vi "input.vi"(2 "位数(2)":i32=2, 3 "in":dbl=1.2345) -> (0 "out":dbl format="%.6f", 1 "值改变?":bool)   [LabVIEW 2018]
panel:
  in  "ESC":bool
  in  "C":bool
  in  "字符串":string
  in  ".":bool
  in  "0":bool
  in  "-":bool
  in  "bk":bool
  in  "en":bool
  in  "3":bool
  in  "2":bool
  in  "1":bool
  in  "6":bool
  in  "5":bool
  in  "4":bool
  in  "9":bool
  in  "8":bool
  in  "7":bool
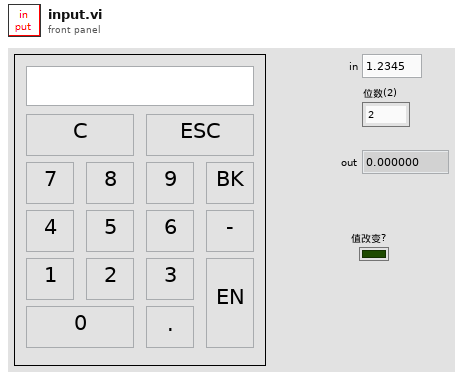
[diagram p1: front panel]
types:
  T1 = enum8{"Enabled", "Disabled", "Disabled and Grayed Out"}
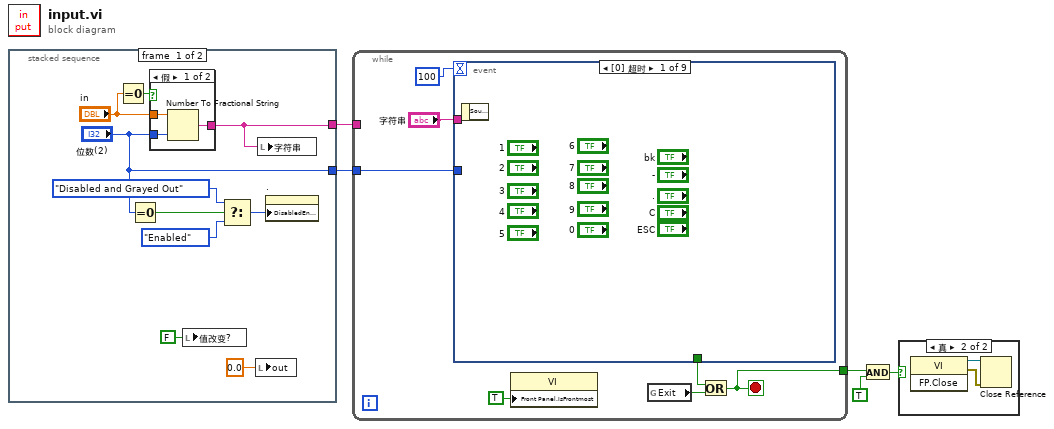
[diagram p0: block diagram]
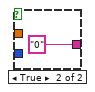
[diagram p2: hidden frame]
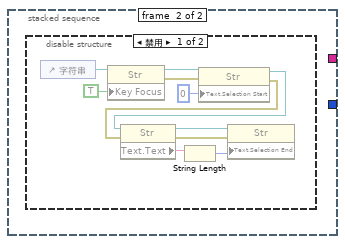
[diagram p3: hidden frame]
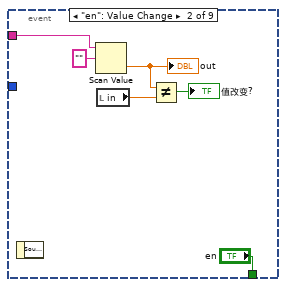
[diagram p6: hidden frame]
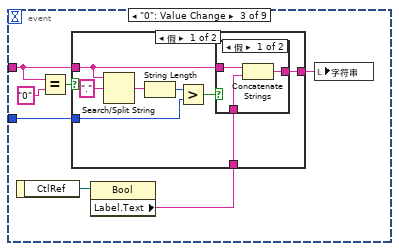
[diagram p7: hidden frame]
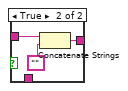
[diagram p8: hidden frame]
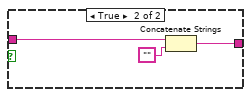
[diagram p9: hidden frame]
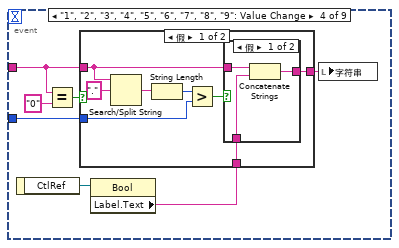
[diagram p10: hidden frame]
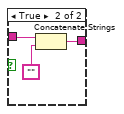
[diagram p11: hidden frame]
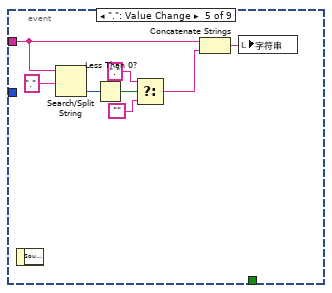
[diagram p13: hidden frame]
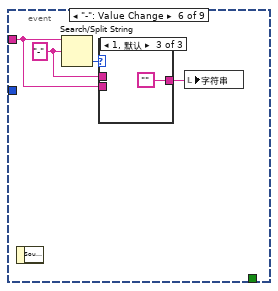
[diagram p14: hidden frame]
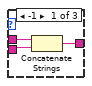
[diagram p15: hidden frame]
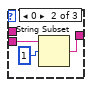
[diagram p16: hidden frame]
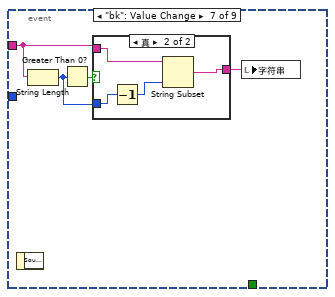
[diagram p17: hidden frame]
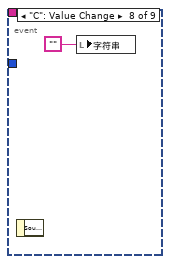
[diagram p19: hidden frame]
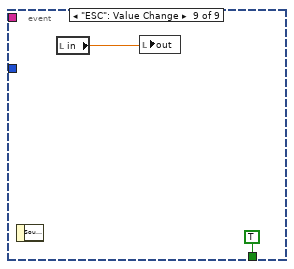
[diagram p20: hidden frame]
diagram:
  n1 = stacked-sequence {
    tunnel: [w15 _] -> w5
    tunnel: ["位数(2)" _] -> w1
    frame #0 {
      n2 = Equal To 0?(x="in") -> (x = 0?=w13:bool)
      n3 = Equal To 0?(x="位数(2)") -> (x = 0?=w9:bool)
      n4 = case shown="假" w13 {
        tunnel: "in" -> [w18 _]
        tunnel: [w17 "0"] -> w15
        tunnel: "位数(2)" -> [w16 _]
        frame False {
          n5 = Number To Fractional String(number=w18, precision (6)=w16) -> (F-format string=w17:string)  [unwired: 2 in]
        }
        frame True {
        }
      }
      n6 = local write "值改变?"(FALSE ("值改变")) -> ()
      n7 = Select(t=T1."Disabled and Grayed Out" ("禁用"), s=w9, f=T1."Enabled" ("禁用")) -> (s? t:f=w8:T1)
      n8 = local write "out"(0.0) -> ()
      n9 = local write "字符串"(w15) -> ()
      n10 = property on="." class="Bool"("DisabledEnum"=w8) -> ()  [unwired: 2 in, 2 out]
    }
    frame #1 {
      n11 = disable-structure shown="禁用" {
        frame Disabled {
          n12 = control-ref of="字符串"() -> (w28:refnum<vi>)
          n13 = property class="Str"(reference=w28, "Key Focus"=TRUE ("键选中")) -> (reference out=w25:refnum<vi>, error out=w24:errorcluster)  [unwired: 1 in]
          n14 = property class="Str"(reference=w25, error in=w24, "Text.Selection Start"=u32 0 ("文本.选择区域:起始")) -> (reference out=w21:refnum<vi>, error out=w22:errorcluster)
          n15 = property class="Str"(reference=w21, error in=w22) -> (reference out=w29:refnum<vi>, error out=w20:errorcluster, "Text.Text"=w30:string)
          n16 = String Length(string=w30) -> (length=w26:i32)
          n17 = property class="Str"(reference=w29, error in=w20, "Text.Selection End"=w26) -> ()  [unwired: 2 out]
        }
        frame Enabled {
        }
      }
    }
  }
  n18 = while {
    tunnel: [w34] -> w4
    tunnel: w5 -> [_]
    tunnel: w1 -> [w31]
    stop <- w34 stop-if-true
    n19 = event shown="[0] 超时" {
      selector: _ -> [_ _ _ _ _ _ _ _ _]
      dyn-events: _ -> [_ _ _ _ _ _ _ _ _]
      timeout: 100 -> [_ _ _ _ _ _ _ _ _]
      tunnel: [_ "en" _ _ _ _ _ _ TRUE ("en")] -> w33
      tunnel: "字符串" -> [_ w42 w49 w69 w96 w99 w110 _ _]
      tunnel: w31 -> [_ _ w45 w68 _ _ _ _ _]
      event Timeout {
        n20 = event-data() -> ()  [unwired: 1 in, 1 out]
      }
      event "en": Value Change {
        n21 = event-data() -> ()  [unwired: 1 in, 1 out]
        n22 = Scan Value(string=w42, format string="" ("格式字符串")) -> (value=w40:dbl)  [unwired: 1 in, 1 out]
        "out" <- w40
        n23 = local read "in"() -> (w39:dbl)
        n24 = Not Equal?(x=w40, y=w39) -> (x != y?=→"值改变?":bool)
      }
      event "0": Value Change {
        n25 = event-data() -> ("CtlRef"=w46:refnum<vi>)  [unwired: 1 in]
        n26 = Equal?(x=w49, y="0") -> (x = y?=w47:bool)
        n27 = property class="Bool"(reference=w46) -> ("Label.Text"=w44:string)  [unwired: 1 in, 2 out]
        n28 = case shown="假" w47 {
          tunnel: w49 -> [w52 w67]
          tunnel: [w53 w66] -> w48
          tunnel: w45 -> [w55 _]
          tunnel: w44 -> [w51 _]
          frame False {
            n29 = Search/Split String(string=w52, search string/char (-)="." ("搜索字符串/字符(-)")) -> (match + rest of string=w57:string)  [unwired: 1 in, 2 out]
            n30 = String Length(string=w57) -> (length=w56:i32)
            n31 = Greater?(x=w56, y=w55) -> (0:w54:bool)
            n32 = case shown="假" w54 {
              tunnel: [w61 w63] -> w53
              tunnel: w52 -> [w60 w62]
              tunnel: w51 -> [w59 _]
              frame False {
                n33 = Concatenate Strings(w60, w59) -> (w61:string)
              }
              frame True {
                n34 = Concatenate Strings(w62, "") -> (w63:string)
              }
            }
          }
          frame True {
            n35 = Concatenate Strings(w67, "") -> (w66:string)
          }
        }
        n36 = local write "字符串"(w48) -> ()
      }
      event "1", "2", "3", "4", "5", "6", "7", "8", "9": Value Change {
        n37 = event-data() -> ("CtlRef"=w74:refnum<vi>)  [unwired: 1 in]
        n38 = Equal?(x=w69, y="0") -> (x = y?=w72:bool)
        n39 = property class="Bool"(reference=w74) -> ("Label.Text"=w71:string)  [unwired: 1 in, 2 out]
        n40 = case shown="假" w72 {
          tunnel: w71 -> [w75 w89]
          tunnel: [w82 w89] -> w70
          tunnel: w69 -> [w81 _]
          tunnel: w68 -> [w77 _]
          frame False {
            n41 = Search/Split String(string=w81, search string/char (-)="." ("搜索字符串/字符(-)")) -> (match + rest of string=w79:string)  [unwired: 1 in, 2 out]
            n42 = String Length(string=w79) -> (length=w78:i32)
            n43 = Greater?(x=w78, y=w77) -> (0:w76:bool)
            n44 = case shown="假" w76 {
              tunnel: [w85 w88] -> w82
              tunnel: w81 -> [w84 w87]
              tunnel: w75 -> [w83 _]
              frame False {
                n45 = Concatenate Strings(w84, w83) -> (w85:string)
              }
              frame True {
                n46 = Concatenate Strings(w87, "") -> (w88:string)
              }
            }
          }
          frame True {
          }
        }
        n47 = local write "字符串"(w70) -> ()
      }
      event ".": Value Change {
        n48 = event-data() -> ()  [unwired: 1 in, 1 out]
        n49 = Search/Split String(string=w96, search string/char (-)=".") -> (offset of match=w94:i32)  [unwired: 1 in, 2 out]
        n50 = Less Than 0?(x=w94) -> (x < 0?=w93:bool)
        n51 = Select(t=".", s=w93, f="") -> (s? t:f=w91:string)
        n52 = Concatenate Strings(w96, w91) -> (w97:string)
        n53 = local write "字符串"(w97) -> ()
      }
      event "-": Value Change {
        w100 = "-" ("搜索字符串/字符(-)")
        n54 = event-data() -> ()  [unwired: 1 in, 1 out]
        n55 = Search/Split String(string=w99, search string/char (-)=w100) -> (offset of match=w101:i32)  [unwired: 1 in, 2 out]
        n56 = case shown="1, 默认" w101 {
          tunnel: w100 -> [w104 _ _]
          tunnel: w99 -> [w103 w107 _]
          tunnel: [w102 w105 ""] -> w98
          frame -1 {
            n57 = Concatenate Strings(w104, w103) -> (w102:string)
          }
          frame 0 {
            n58 = String Subset(string=w107, offset (0)=1 ("偏移量(0)")) -> (substring=w105:string)  [unwired: 1 in]
          }
          frame 1, Default {
          }
        }
        n59 = local write "字符串"(w98) -> ()
      }
      event "bk": Value Change {
        n60 = event-data() -> ()  [unwired: 1 in, 1 out]
        n61 = String Length(string=w110) -> (length=w109:i32)
        n62 = Greater Than 0?(x=w109) -> (x > 0?=w111:bool)
        n63 = case shown="真" w111 {
          tunnel: [w113 w117] -> w112
          tunnel: w110 -> [w113 w116]
          tunnel: w109 -> [_ w115]
          frame False {
          }
          frame True {
            n64 = Decrement(x=w115) -> (x-1=w114:i32)
            n65 = String Subset(string=w116, length (rest)=w114) -> (substring=w117:string)  [unwired: 1 in]
          }
        }
        n66 = local write "字符串"(w112) -> ()
      }
      event "C": Value Change {
        n67 = event-data() -> ()  [unwired: 1 in, 1 out]
        n68 = local write "字符串"("") -> ()
      }
      event "ESC": Value Change {
        n69 = event-data() -> ()  [unwired: 1 in, 1 out]
        n70 = local read "in"() -> (w120:dbl)
        n71 = local write "out"(w120) -> ()
      }
    }
    n72 = property class="VI"("Front Panel.IsFrontmost"=TRUE) -> ()  [unwired: 2 in, 2 out]
    n73 = global read "全局 1.vi" "Exit"() -> (w32:bool)
    n74 = Or(x=w33, y=w32) -> (x .or. y?=w34:bool)
  }
  n75 = And(x=w4, y=TRUE) -> (x .and. y?=w3:bool)
  n76 = case shown="真" w3 {
    frame False {
    }
    frame True {
      n77 = invoke class="VI" method="FP.Close"() -> (reference out=w121:refnum<vi>, error out=w122:errorcluster)  [unwired: 3 in, 1 out]
      n78 = Close Reference(reference=w121, error in (no error)=w122) -> ()  [unwired: 1 out]
    }
  }
